vi "setNewItem.vi"(8 "error in (no error)":errorcluster, 9 "dim":i32, 10 "index":i32, 11 "reference in":refnum<class "trackingNotification.lvclass">) -> (0 "error out":errorcluster, 3 "reference out":refnum<class "trackingNotification.lvclass">)   [LabVIEW 2016, in "trackingNotification.lvclass"]
uses:
  trackingNotification.lvclass
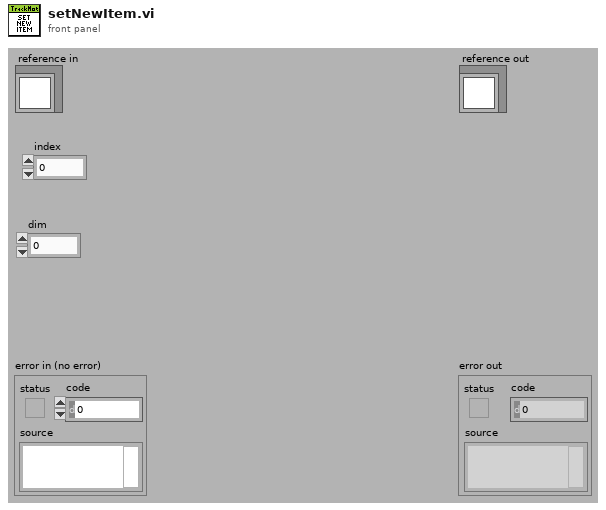
[diagram p1: front panel]
types:
  T1 = typedef "trackingNotification.lvclass/ObjectAttributesRef.ctl" = refnum<data-value>
  T2 = typedef "trackingNotification.lvclass/ObjectAttributes.ctl" = cluster{"MyAttribute":dbl, "index_parts_expired":i32[], "data":string[][]}
  T3 = typedef "trackingNotification.lvclass/ClassAttributesRef.ctl" = refnum<data-value>
  T4 = typedef "trackingNotification.lvclass/ClassAttributes.ctl" = cluster{"Dummy":bool, "tracking_notification_refs":refnum<class "trackingNotification.lvclass">[]}
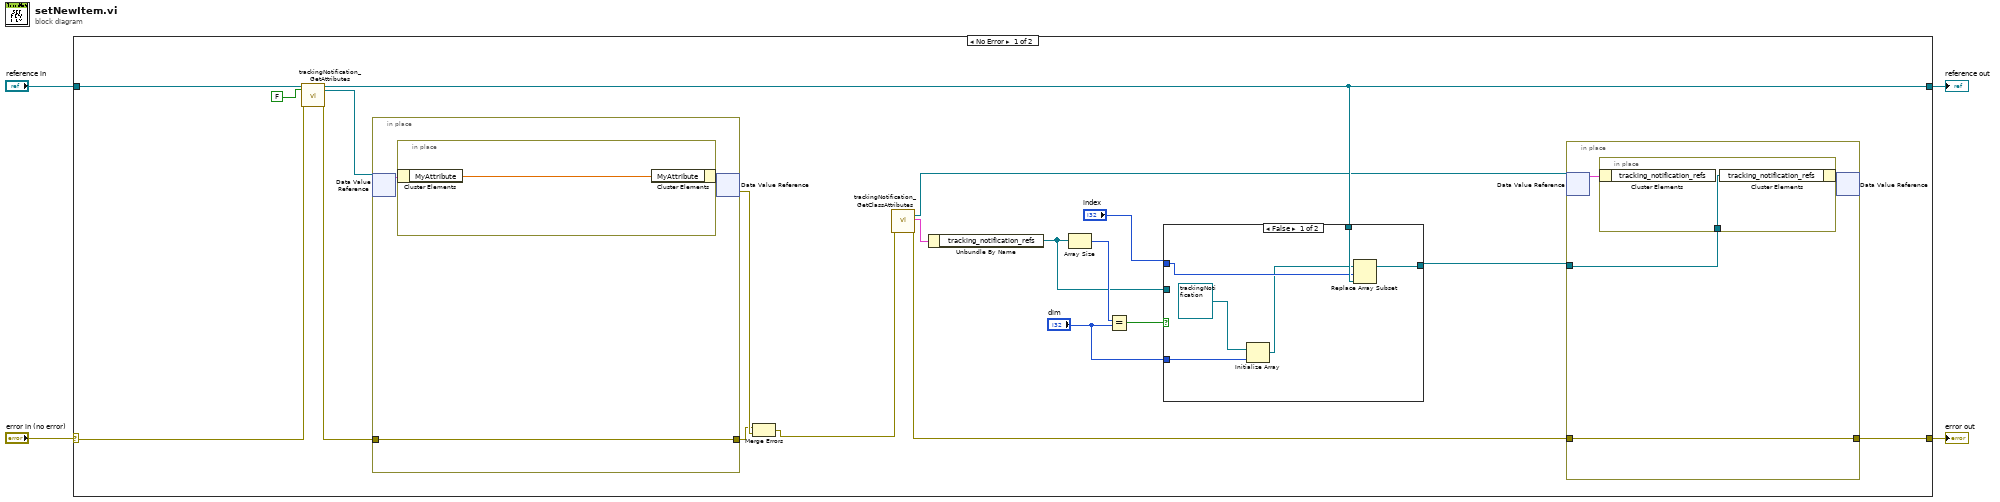
[diagram p0: block diagram]
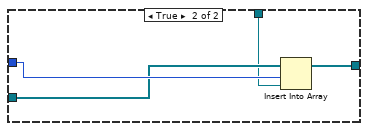
[diagram p2: hidden frame]
diagram:
  n1 = case shown="No Error" "error in (no error)" {
    selector: "error in (no error)" -> [w19 w44]
    tunnel: [w10 w44] -> w3
    tunnel: [w13 w43] -> w1
    tunnel: "reference in" -> [w21 w43]
    frame No Error {
      n2 = call "trackingNotification_GetAttributes.vi"("reference in"=w21, "return data? (T)"=FALSE, "error in (no error)"=w19) -> ("reference out"=w13:refnum<class "trackingNotification.lvclass">, "attributes ref"=w17:T1, "error out"=w18:errorcluster)  [unwired: 13 in, 1 out]
      n3 = in-place {
        in-place-border: w18 -> [w39]
        in-place-border: [w39] -> w22
        n4 = in-place-dvr #1(w17) -> (w40:T2)  [unwired: 1 out]
        n5 = in-place {
          n6 = in-place-cluster #2(w40) -> ("MyAttribute"=w42:dbl)
          n7 = in-place-cluster #2("MyAttribute"=w42) -> (w41:T2)
        }
        n8 = in-place-dvr #1(w41) -> (w23:errorcluster)  [unwired: 1 out]
      }
      n9 = Merge Errors(w22, w23) -> (w7:errorcluster)
      n10 = call "trackingNotification_GetClassAttributes.vi"("error in (no error)"=w7) -> ("class attributes ref"=w9:T3, "class attributes"=w16:T4, "error out"=w11:errorcluster)  [unwired: 15 in, 1 out]
      n11 = Unbundle By Name(w16) -> ("tracking_notification_refs"=w12:refnum<class "trackingNotification.lvclass">[])
      n12 = Array Size(array=w12) -> (size(s)=w15:i32)
      n13 = Equal?(x=w15, y="dim") -> (x = y?=w14:bool)
      n14 = case shown="False" w14 {
        tunnel: "index" -> [w33 w38]
        tunnel: w13 -> [w34 w35]
        tunnel: w12 -> [_ w37]
        tunnel: [w31 w36] -> w8
        tunnel: "dim" -> [w29 _]
        frame False {
          n15 = Initialize Array(refnum<class "trackingNotification.lvclass"> refnum ("device.lvclass"), w29) -> (w32:refnum<class "trackingNotification.lvclass">[])
          n16 = Replace Array Subset(array=w32, new element=w34, index=w33) -> (w31:refnum<class "trackingNotification.lvclass">[])
        }
        frame True {
          n17 = Insert Into Array(array=w37, index=w38, new element=w35) -> (w36:refnum<class "trackingNotification.lvclass">[])
        }
      }
      n18 = in-place {
        in-place-border: w11 -> [w25]
        in-place-border: [w25] -> w10
        in-place-border: w8 -> [w24]
        n19 = in-place-dvr #3(w9) -> (w26:T4)  [unwired: 1 out]
        n20 = in-place {
          in-place-border: w24 -> [w28]
          n21 = in-place-cluster #4(w26) -> ()  [unwired: 1 out]
          n22 = in-place-cluster #4("tracking_notification_refs"=w28) -> (w27:T4)
        }
        n23 = in-place-dvr #3(w27) -> ()  [unwired: 2 out]
      }
    }
    frame Error {
    }
  }
  "error out" <- w3
  "reference out" <- w1
